vi "Stopwatch.vi"(5 "error in (no error)":errorcluster) -> (1 "error out":errorcluster, 2 "millisecond timer value":u32)   [LabVIEW 2015]
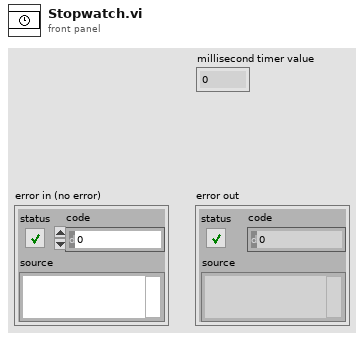
[diagram p1: front panel]
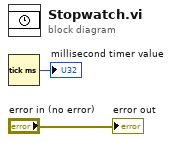
[diagram p0: block diagram]
diagram:
  n1 = Tick Count (ms)() -> (millisecond timer value=→"millisecond timer value":u32)
  "error out" <- "error in (no error)"
